vi "Vbias V To Word.vi"(0 "VB":dbl) -> (4 "Vbias Word":u8 format="%08b")   [LabVIEW 2020]
uses:
  <vilib>/gmath/NI_Gmath.lvlib
  9b3954db-bb76-4350-b219-fa9f862701d0.vi
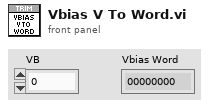
[diagram p1: front panel]
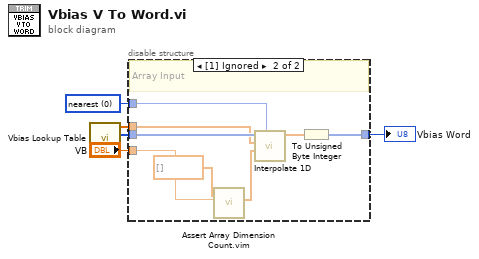
[diagram p0: block diagram]
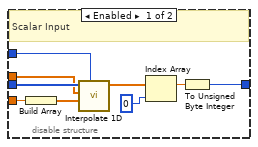
[diagram p2: hidden frame]
diagram:
  w5 = 0 items=["nearest", "linear", "spline", "cubic Hermite", "Lagrange"] ("method")
  n1 = call "Vbias Lookup Table.vi"() -> ("ROUT<7:5>"=w4:u8[], "VB(V)"=w3:dbl[])  [unwired: 10 in]
  n2 = disable-structure shown="[1] Ignored" {
    disable-tunnel: w5 -> [w14 w22]
    disable-tunnel: w4 -> [w13 w21]
    disable-tunnel: w3 -> [w11 w19]
    disable-tunnel: [w10 w18] -> w2
    disable-tunnel: "VB" -> [w9 w16]
    frame Enabled {
      # "Scalar Input"
      n3 = Build Array(w9) -> (w8:dbl[])
      n4 = call <vilib>:"Interpolate 1D.vi"("method"=w14, "xi"=w8, "X"=w11, "Y"=w13) -> ("yi"=w12:dbl[])  [unwired: 5 in, 2 out]
      n5 = Index Array(array=w12, index=0) -> (element=w7:dbl)
      n6 = To Unsigned Byte Integer(number=w7) -> (unsigned 8bit integer=w10:u8)
    }
    frame Disabled {
      # "Array Input"
      n7 = call "Assert Array Dimension Count.vim"("array type"=dbl[] [], "value in"=w16) -> ("value out"=w15:dbl[])  [unwired: 7 in]
      n8 = call <vilib>:"Interpolate 1D.vi"("method"=w22, "xi"=w15, "X"=w19, "Y"=w21) -> ("yi"=w20:dbl[])  [unwired: 5 in, 2 out]
      n9 = To Unsigned Byte Integer(number=w20) -> (unsigned 8bit integer=w18:u8[])
    }
  }
  "Vbias Word" <- w2
